vi "sıcaklık.vi"() -> ()   [LabVIEW 2018]
uses:
  <vilib>/MakerHub/LINX/Public/Peripherals/Analog/Analog Read 1 Chan.vi
  <vilib>/MakerHub/LINX/Public/Peripherals/Analog/Analog Read N Chans.vi
  <vilib>/MakerHub/LINX/Private/Local IO/LinxAnalogRead.vi
  <vilib>/MakerHub/LINX/Public/Utilities/Check Channel.vi
  <vilib>/MakerHub/LINX/Public/Utilities/Open Serial.vi
  <vilib>/MakerHub/LINX/Private/Utilties/Generate Error.vi
  <vilib>/MakerHub/LINX/LMH-LINX.lvlib
panel:
  out "Led":bool
  out "Thermometer":dbl(slide) scale=0.0..100.0
  out "Sicaklik":dbl
  in  "Serial Port":refnum<visa-resource-name>="N/A"
  in  "Analog Channel 3":u8
  in  "stop":bool
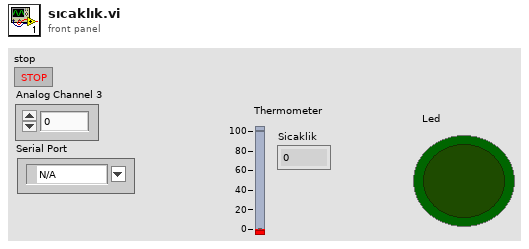
[diagram p1: front panel]
types:
  T1 = typedef "LMH-LINX.lvlib/LINX Ref.ctl" = cluster{"IO":T2, "Interface":T3, "LINX Device Config":T4}
  T2 = typedef "LMH-LINX.lvlib/Platform.ctl" = enum16{"Remote", "Local"}
  T3 = typedef "LMH-LINX.lvlib/Interface.ctl" = enum16{"Serial", "TCP"}
  T4 = typedef "LMH-LINX.lvlib/Device.lvlib/LINX Device Config.ctl" = cluster{"Interface":T3, "COM Port":refnum<visa-resource-name>, "TCP Configuration":T5, "Device Family":u8, "Device ID":u8, "Device Name":string, "TCP Ref":refnum<k5>, "Channels":T6}
  T5 = typedef "LMH-LINX.lvlib/Device.lvlib/TCP Config.ctl" = cluster{"IP Address":string, "Port":u16}
  T6 = typedef "LMH-LINX.lvlib/Channels.ctl" = cluster{"DI":u8[], "DO":u8[], "AI":u8[], "AO":u8[], "PWM":u8[], "QE":u8[], "UART":u8[], "I2C 2":u8[], "SPI":u8[], "CAN":u8[], "Servo":u8[], "AI Ref (V)":dbl, "AI Resolution (Bits)":u8, "AO Ref (V)":dbl, "AO Resolution (Bits)":u8}
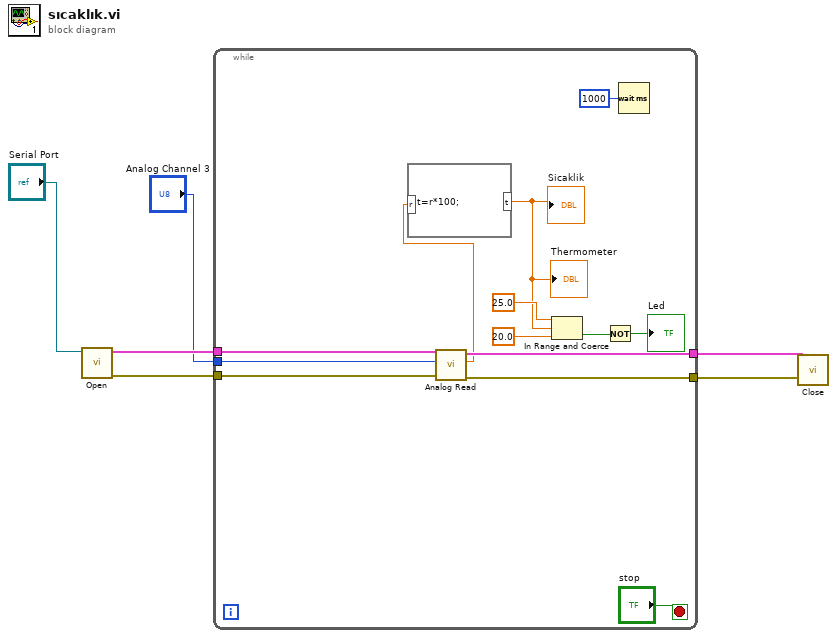
[diagram p0: block diagram]
diagram:
  n1 = call-poly <vilib>:"Open.vi"("Serial Port"="Serial Port") -> ("Error Out"=w6:errorcluster, "LINX Resource"=w4:T1)  [unwired: 8 in, 1 out]
  n2 = while {
    tunnel: w6 -> [w18]
    tunnel: [w17] -> w5
    tunnel: w4 -> [w16]
    tunnel: [w15] -> w3
    tunnel: "Analog Channel 3" -> [w14]
    stop <- "stop" stop-if-true
    n3 = call-poly <vilib>:"Analog Read.vi"("Error In"=w18, "Analog Channel"=w14, "LINX Resource"=w16) -> ("Error Out"=w17:errorcluster, "Voltage"=w13:dbl, "LINX Resource"=w15:T1)  [unwired: 5 in, 1 out]
    n4 = formula code="t=r*100;"("r"=w13) -> ("t"=w10:dbl)
    "Sicaklik" <- w10
    "Thermometer" <- w10
    n5 = In Range and Coerce(upper limit=25.0, x=w10, lower limit=20.0) -> (In Range?=w9:bool)  [unwired: 1 out]
    n6 = Not(x=w9) -> (.not. x?=→"Led":bool)
    n7 = Wait (ms)(milliseconds to wait=u32 1000) -> ()  [unwired: 1 out]
  }
  n8 = call <vilib>:"Close.vi"("Error In"=w5, "LINX Resource"=w3) -> ()  [unwired: 9 in, 1 out]
